vi "CreateStaveMapFromCalibration.vi"() -> ()   [LabVIEW 2016]
uses:
  <vilib>/Utility/file.llb/Write Delimited Spreadsheet (DBL).vi
panel:
  in  "Reports path":path=path "C:/Users/Aerotech/cernbox/BNL/Stave Assembly Records/2017-05-10"
  in  "Code path":path=path "C:/Users/Aerotech/Documents/BNL_ThermomechanicalStave"
  in  "Stereo Angle [mrad]":dbl=40.0 format="%#_13g"
  in  "Build Config":T1={"Tape Type"=enum."Left stereo", "Stave Coordinate System"=enum."Bus Tape", "Module fiducial marker"=enum."Mark C", "N Modules"=13}
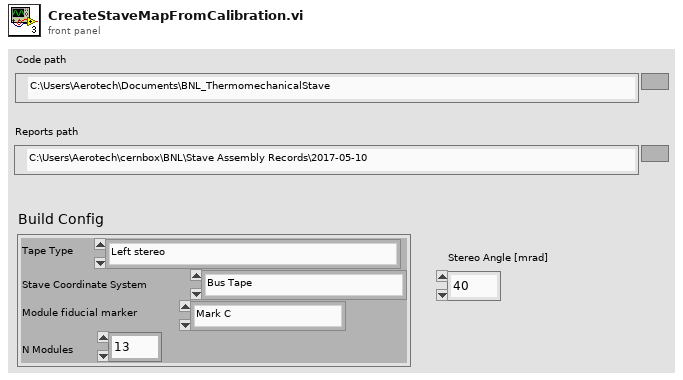
[diagram p1: front panel]
types:
  T1 = cluster{"Tape Type":enum16{"Right stereo", "Left stereo", "Stereo (Sutcliffe NP49-01-100 01-Mar-16)", "Axial (Sutcliffe NP49-01-100 01-Mar-16)"}, "Stave Coordinate System":enum16{"Tooling Pins", "Bus Tape"}, "Module fiducial marker":enum16{"Mark B", "Mark C", "Strip Corner", "Mark I (Slim/17)", "Mark E (Slim/17)", "Mark F (Slim/17)", "Mark G (Slim/17)", "Mark A (12)"}, "N Modules":i32}
  T2 = enum16{"ATLAS07", "ATLAS12", "ATLAS12Slim", "ATLAS17LS"}
  T3 = enum16{"Right stereo", "Left stereo", "Stereo (Sutcliffe NP49-01-100 01-Mar-16)", "Axial (Sutcliffe NP49-01-100 01-Mar-16)"}
  T4 = enum16{"Mark B", "Mark C", "Strip Corner", "Mark I (Slim/17)", "Mark E (Slim/17)", "Mark F (Slim/17)", "Mark G (Slim/17)", "Mark A (12)"}
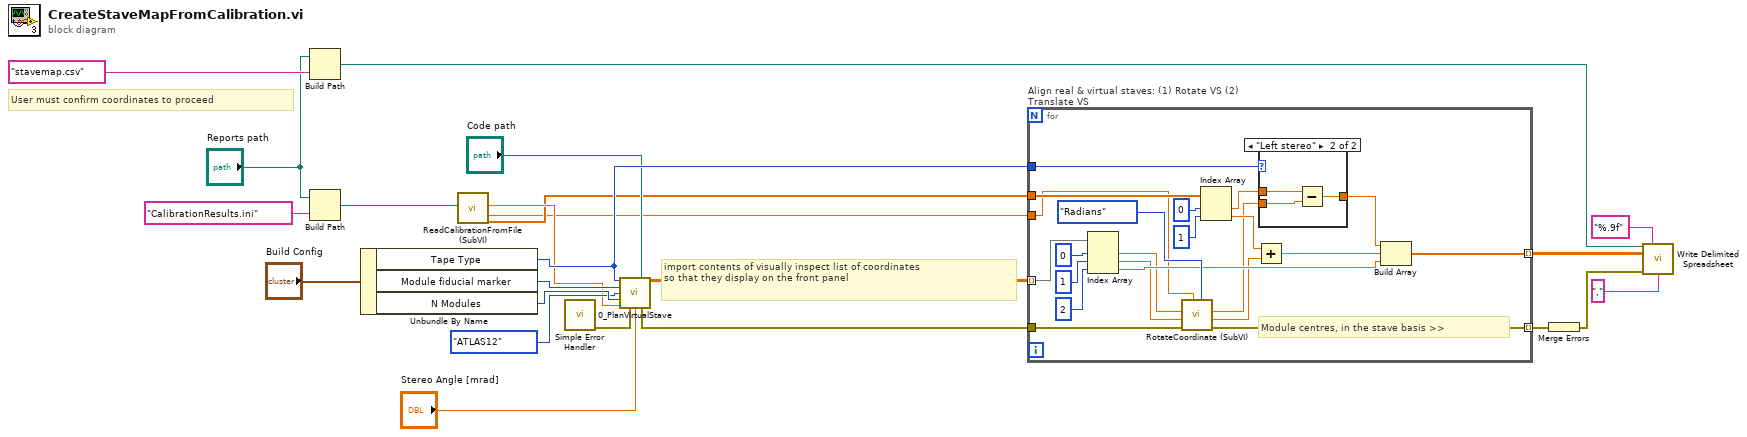
[diagram p0: block diagram]
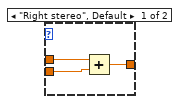
[diagram p2: hidden frame]
diagram:
  # "User must confirm coordinates to proceed"
  # "import contents of visually inspect list of coordinates\nso that they display on the front panel"
  n1 = Build Path(base path="Reports path", name or relative path="stavemap.csv") -> (appended path=w21:path)
  n2 = Build Path(base path="Reports path", name or relative path="CalibrationResults.ini") -> (appended path=w4:path)
  n3 = Unbundle By Name("Build Config") -> ("Tape Type"=w9:T3, "Module fiducial marker"=w12:T4, "N Modules"=w13:i32)
  n4 = call "ReadCalibrationFromFile (SubVI).vi"("Calibration file path"=w4) -> ("CameraWD"=w3:dbl, "Angle"=w1:dbl, "Stave Origin"=w2:dbl[])  [unwired: 12 in, 4 out]
  n5 = call <vilib>:"Simple Error Handler.vi"() -> ("error out"=w15:errorcluster)  [unwired: 5 in, 4 out]
  n6 = call "0_PlanVirtualStave.vi"("Tape Type"=w9, "Code path"="Code path", "Module fiducial marker"=w12, "Sensor Pattern"=T2."ATLAS12", "N Modules"=w13, "Working height [mm]"=w3, "error in (no error)"=w15, "Stereo Angle [mrad]"="Stereo Angle [mrad]") -> ("Stave Basis: Coordinates of Fiducials on Modules"=w17:dbl[][], "error out"=w10:errorcluster)  [unwired: 5 in, 1 out]
  n7 = for "Align real & virtual staves: (1) Rotate VS (2) Translate VS" {
    tunnel: w17 -> [w45] mode=indexing
    tunnel: [w39] -> w23 mode=indexing
    tunnel: [w28] -> w16 mode=indexing
    tunnel: w10 -> [w27]
    tunnel: w9 -> [w26]
    tunnel: w2 -> [w25]
    tunnel: w1 -> [w24]
    # "Module centres, in the stave basis >>"
    n8 = Index Array(array=w45, index #1=0 ("index"), index #2=1 ("index"), index #3=2 ("index")) -> (element #1=w32:dbl, element #2=w29:dbl, element #3=w33:dbl)
    n9 = call "RotateCoordinate (SubVI).vi"("Units"=enum16{"mrad", "Radians", "Degrees"}."Radians", "Angle"=w24, "error in (no error)"=w27, "y"=w29, "x"=w32) -> ("error out"=w28:errorcluster, "y'"=w30:dbl, "x'"=w31:dbl)  [unwired: 4 in]
    n10 = Index Array(array=w25, index #1=0 ("index"), index #2=1 ("index")) -> (element #1=w37:dbl, element #2=w35:dbl)
    n11 = Add(x=w35, y=w30) -> (x+y=w40:dbl)
    n12 = case shown="\"Left stereo\"" w26 {
      tunnel: [w48 w51] -> w41
      tunnel: w37 -> [w47 w50]
      tunnel: w31 -> [w46 w49]
      frame "Right stereo", Default {
        n13 = Add(x=w47, y=w46) -> (x+y=w48:dbl)
      }
      frame "Left stereo" {
        n14 = Subtract(x=w50, y=w49) -> (x-y=w51:dbl)
      }
    }
    n15 = Build Array(w41, w40, w33) -> (w39:dbl[])
  }
  n16 = Merge Errors(w16) -> (w19:errorcluster)
  n17 = call-poly <vilib>:"Write Delimited Spreadsheet.vi"("file path (dialog if empty)"=w21, "format (%.3f)"="%.9f", "2D data"=w23, "error in (no error)"=w19, "delimiter (\\t)"="," ("delimiter (\\t)")) -> ()  [unwired: 9 in, 2 out]
